vi "PanelClose.vi"(0 "vi reference":refnum<vi>) -> ()   [LabVIEW 2014, in "Panels.lvlib"]
uses:
  Panels.lvlib
panel:
  out "error out":errorcluster
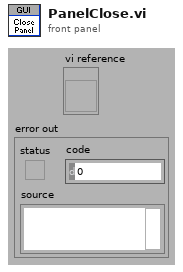
[diagram p1: front panel]
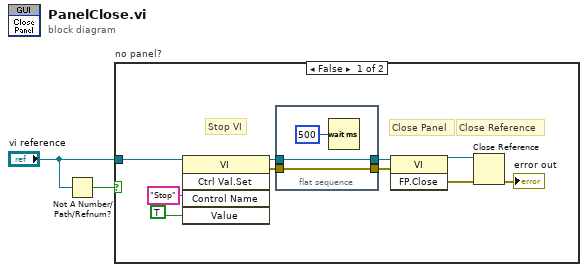
[diagram p0: block diagram]
diagram:
  n1 = Not A Number/Path/Refnum?(number/path/refnum="vi reference") -> (NaN/Path/Refnum?=w1:bool)
  n2 = case "no panel?" shown="False" w1 {
    tunnel: "vi reference" -> [w3 _]
    frame False {
      # "Stop VI"
      # "Close Panel"
      # "Close Reference"
      n3 = invoke class="VI" method="Ctrl Val.Set"(reference=w3, "Control Name"="Stop", "Value"=TRUE) -> (reference out=w9:refnum<vi>, error out=w11:errorcluster)  [unwired: 2 in, 3 out]
      n4 = flat-sequence {
        tunnel: w9 -> [w15]
        tunnel: [w15] -> w10
        tunnel: [w14] -> w12
        tunnel: w11 -> [w14]
        frame #0 {
          n5 = Wait (ms)(milliseconds to wait=u32 500) -> ()  [unwired: 1 out]
        }
      }
      n6 = invoke class="VI" method="FP.Close"(reference=w10, error in=w12) -> (reference out=w6:refnum<vi>, error out=w5:errorcluster)  [unwired: 1 in, 1 out]
      n7 = Close Reference(reference=w6, error in (no error)=w5) -> (error out=→"error out":errorcluster)
    }
    frame True {
    }
  }
